vi "Auto_PID_Drive.vi"(5 "Turning_PID_Enable":bool, 6 "dt (s)":dbl=10.0 format="%.3f", 7 "Turning_Setpoint":dbl, 8 "Yaw":dbl=-13.119872265000097, 9 "Turning":dbl, 10 "Power":dbl) -> (2 "Turning":dbl, 3 "Power":dbl)   [LabVIEW 2015]
uses:
  <vilib>/Rock Robotics/Network Tables/NT Read Number.vi
  <vilib>/Rock Robotics/Network Tables/NT Write Number.vi
  <vilib>/addons/control/pid/pid.llb/PID (DBL).vi
  <vilib>/addons/control/pid/NI_PID_pid.lvlib
panel:
  out "Error":dbl
  out "Waveform Chart 2":dbl(graph)
  out "Waveform Chart":cluster{"Turning_Setpoint":dbl, "Yaw":dbl}(graph)={"Turning_Setpoint"=0.0, "Yaw"=-13.119872265000097}
  in  "PID Gains":T1={"proportional gain (Kc)"=0.03, "integral time (Ti, min)"=1.0, "derivative time (Td, min)"=0.0}
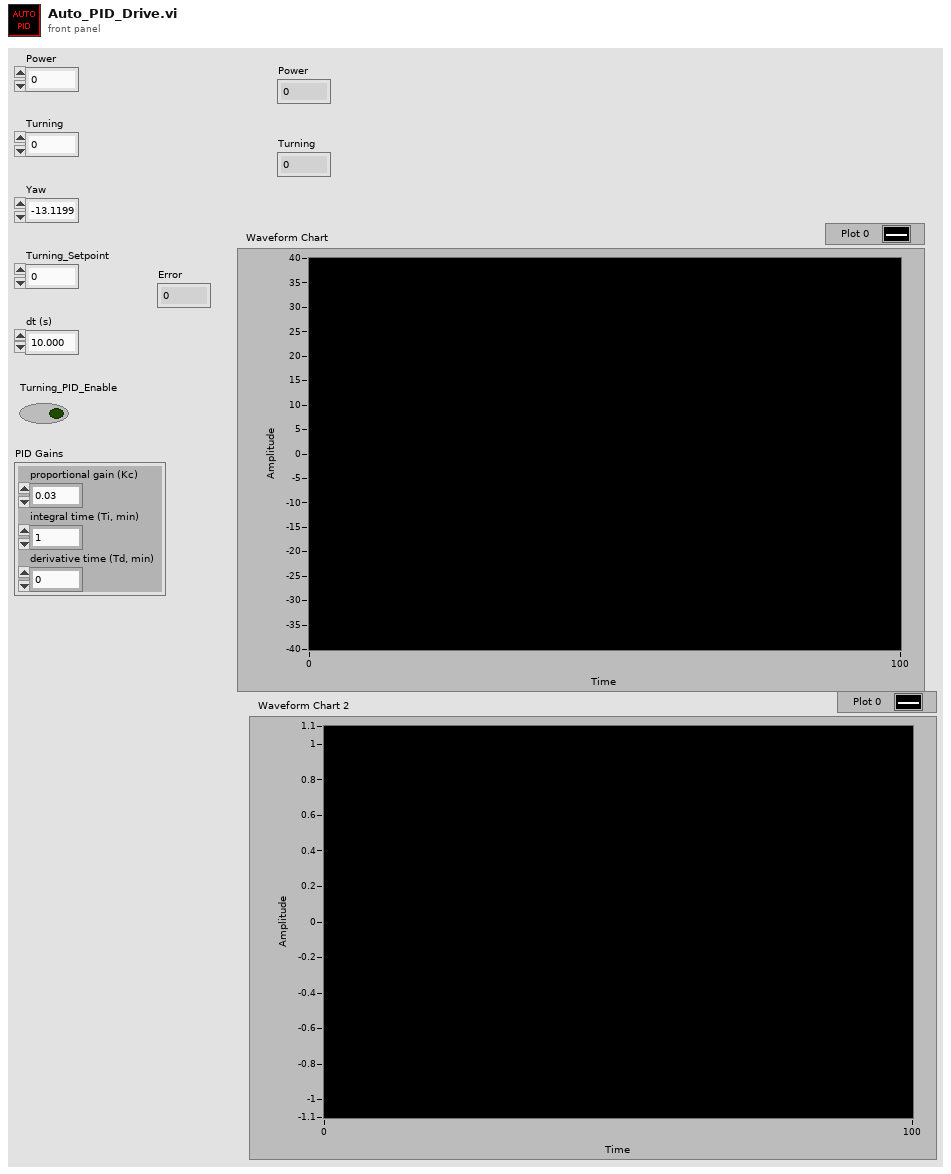
[diagram p1: front panel]
types:
  T1 = cluster{"proportional gain (Kc)":dbl, "integral time (Ti, min)":dbl, "derivative time (Td, min)":dbl}
  T2 = cluster{"Power":dbl, "Yaw":dbl, "Turning_PID_Enable":bool, "Turning":dbl, "Turning_Setpoint":dbl, "PID Gains":cluster{"proportional gain (Kc)":dbl, "integral time (Ti, min)":dbl, "derivative time (Td, min)":dbl}, "dt (s)":dbl}
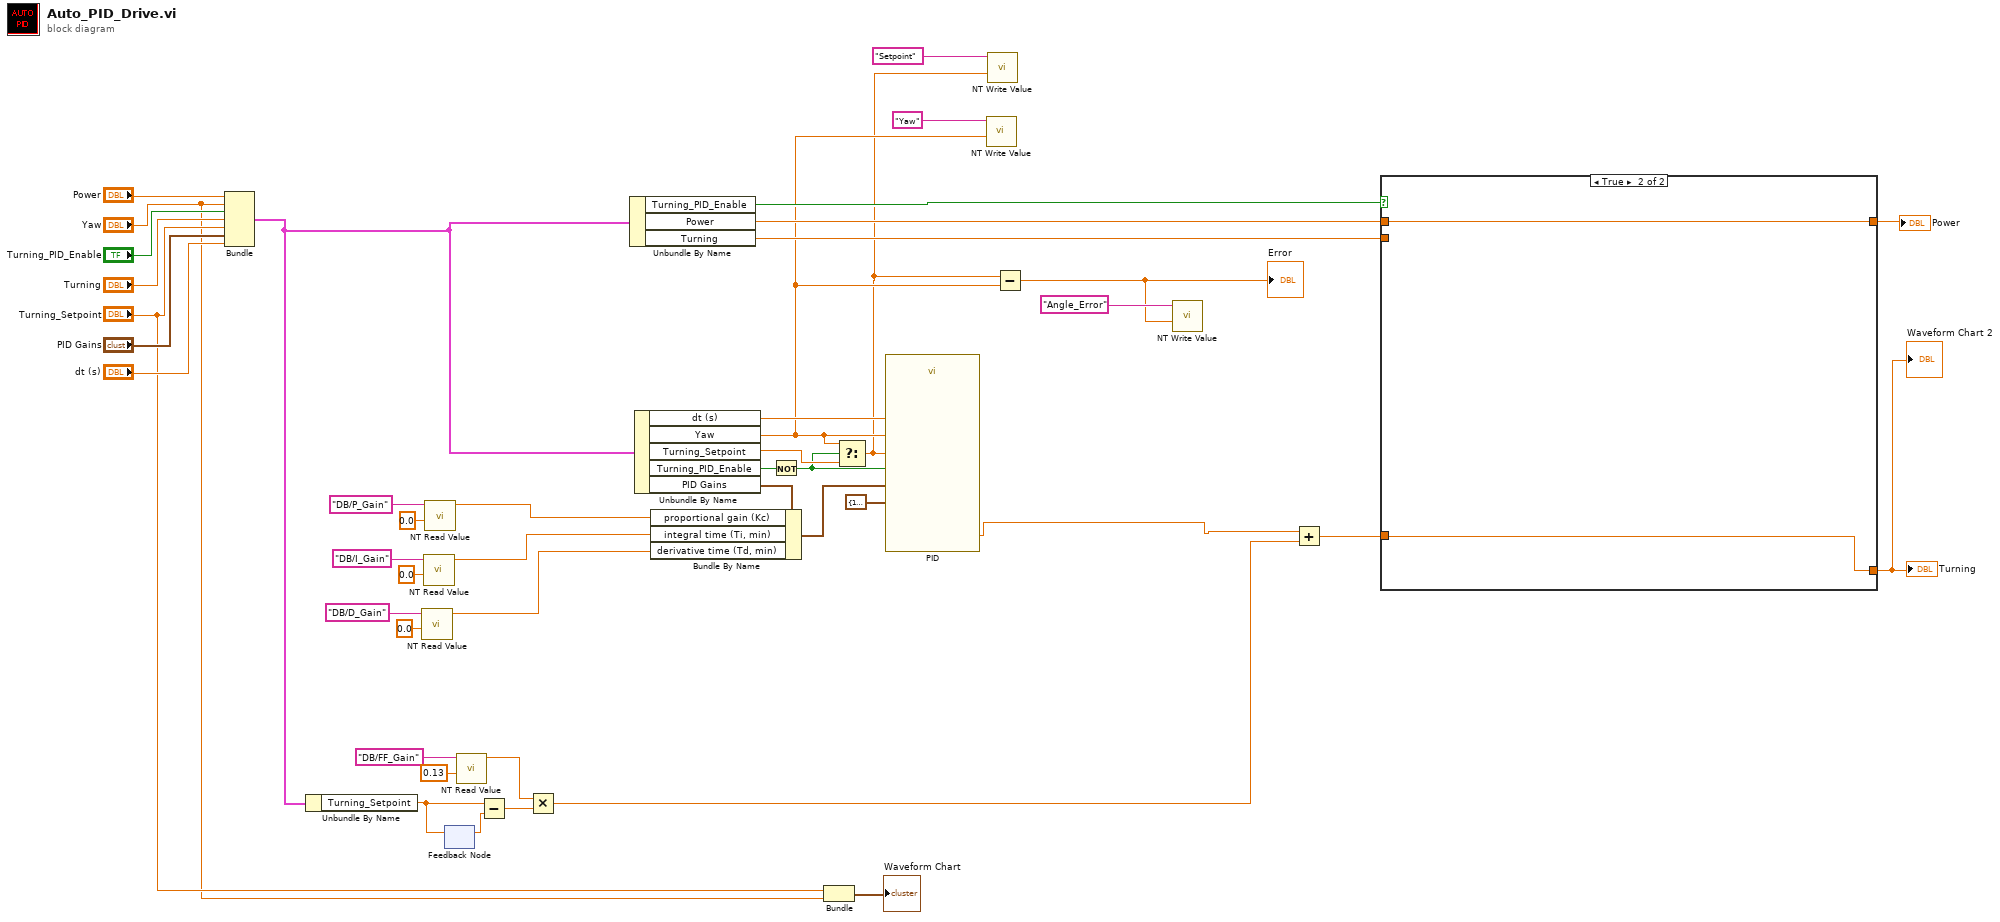
[diagram p0: block diagram]
diagram:
  n1 = Bundle("Power"="Power", "Yaw"="Yaw", "Turning_PID_Enable"="Turning_PID_Enable", "Turning"="Turning", "Turning_Setpoint"="Turning_Setpoint", "PID Gains"="PID Gains", "dt (s)"="dt (s)") -> (w31:T2)  [unwired: 1 in]
  n2 = Unbundle By Name(w31) -> ("Turning_Setpoint"=w34:dbl)
  n3 = call-poly <vilib>:"NT Read Value.vi"("Default Value"=0.0, "Name"="DB/D_Gain" ("refnum name")) -> ("Numeric"=w11:dbl)  [unwired: 8 in, 1 out]
  n4 = call-poly <vilib>:"NT Read Value.vi"("Default Value"=0.0, "Name"="DB/I_Gain" ("refnum name")) -> ("Numeric"=w12:dbl)  [unwired: 8 in, 1 out]
  n5 = call-poly <vilib>:"NT Read Value.vi"("Default Value"=0.0, "Name"="DB/P_Gain" ("refnum name")) -> ("Numeric"=w13:dbl)  [unwired: 8 in, 1 out]
  n6 = feedback-in #1(w34) -> ()
  n7 = feedback #1() -> (w33:dbl)  [unwired: 1 in]
  n8 = call-poly <vilib>:"NT Read Value.vi"("Default Value"=0.13, "Name"="DB/FF_Gain" ("refnum name")) -> ("Numeric"=w19:dbl)  [unwired: 8 in, 1 out]
  n9 = Subtract(x=w34, y=w33) -> (x-y=w32:dbl)
  n10 = Multiply(x=w19, y=w32) -> (x*y=w27:dbl)
  n11 = Unbundle By Name(w31) -> ("Turning_PID_Enable"=w30:bool, "Power"=w35:dbl, "Turning"=w41:dbl)
  n12 = Unbundle By Name(w31) -> ("dt (s)"=w26:dbl, "Yaw"=w5:dbl, "Turning_Setpoint"=w23:dbl, "Turning_PID_Enable"=w25:bool, "PID Gains"=w2:T1)
  n13 = Bundle By Name(cluster=w2, "proportional gain (Kc)"=w13, "integral time (Ti, min)"=w12, "derivative time (Td, min)"=w11) -> (w1:T1)
  n14 = Not(x=w25) -> (.not. x?=w22:bool)
  n15 = Bundle("Turning_Setpoint"="Turning_Setpoint", "Yaw"="Yaw") -> (→"Waveform Chart":cluster{"Turning_Setpoint":dbl, "Yaw":dbl})  [unwired: 1 in]
  n16 = Select(t=w5, s=w22, f=w23) -> (s? t:f=w4:dbl)
  n17 = call-poly <vilib>:"PID.vi"("reinitialize? (F)"=w22, "output range"=cluster{"output high":dbl, "output low":dbl} {"output high"=1.0, "output low"=-1.0}, "dt (s)"=w26, "PID gains"=w1, "process variable"=w5, "setpoint"=w4) -> ("output"=w3:dbl)  [unwired: 4 in, 1 out]
  n18 = call-poly <vilib>:"NT Write Value.vi"("Numeric"=w5, "Name"="Yaw") -> ()  [unwired: 9 in, 1 out]
  n19 = call-poly <vilib>:"NT Write Value.vi"("Numeric"=w4, "Name"="Setpoint") -> ()  [unwired: 9 in, 1 out]
  n20 = Subtract(x=w4, y=w5) -> (x-y=w9:dbl)
  "Error" <- w9
  n21 = call-poly <vilib>:"NT Write Value.vi"("Numeric"=w9, "Name"="Angle_Error") -> ()  [unwired: 9 in, 1 out]
  n22 = Add(x=w3, y=w27) -> (x+y=w24:dbl)
  n23 = case shown="True" w30 {
    tunnel: w35 -> [w47 w49]
    tunnel: w41 -> [w46 _]
    tunnel: [w47 w49] -> w40
    tunnel: [w46 w48] -> w29
    tunnel: w24 -> [_ w48]
    frame False {
    }
    frame True {
    }
  }
  "Power" <- w40
  "Turning" <- w29
  "Waveform Chart 2" <- w29
